vi "Test To Report Entry.vi"(8 "error in (no error)":errorcluster, 10 "Test Node":T1) -> (0 "error out":errorcluster, 2 "String":string)   [LabVIEW 2013, in "Caraya.lvlib" / "Test Report.Event.lvclass"]
uses:
  Test Report.Event.lvclass
  Test Result/Test Node (Extended).ctl
  Test Result/Test Registration Data.ctl
  Test Report/Test Report.lvclass
  Test Result/Test Result.lvclass
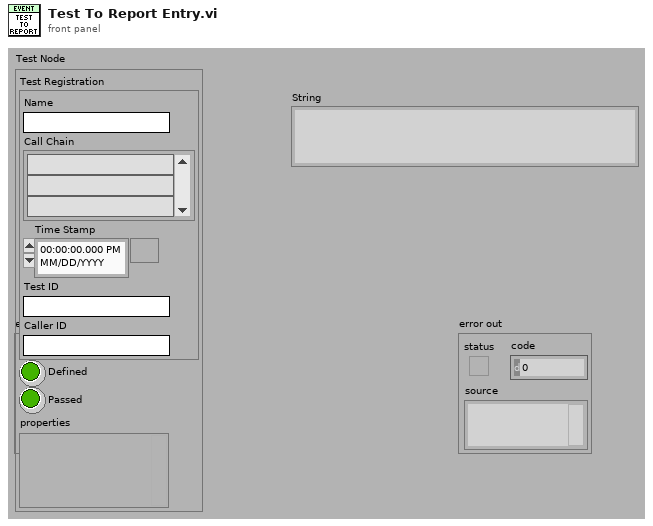
[diagram p1: front panel]
types:
  T1 = typedef "Caraya.lvlib/Test Result.lvclass/Test Node (Extended).ctl" = cluster{"Test Registration":T2, "Defined":bool, "Passed":bool, "properties":variant}
  T2 = typedef "Caraya.lvlib/Test Result.lvclass/Test Registration Data.ctl" = cluster{"Name":string, "Call Chain":string[], "Time Stamp":timestamp, "Test ID":string, "Caller ID":string}
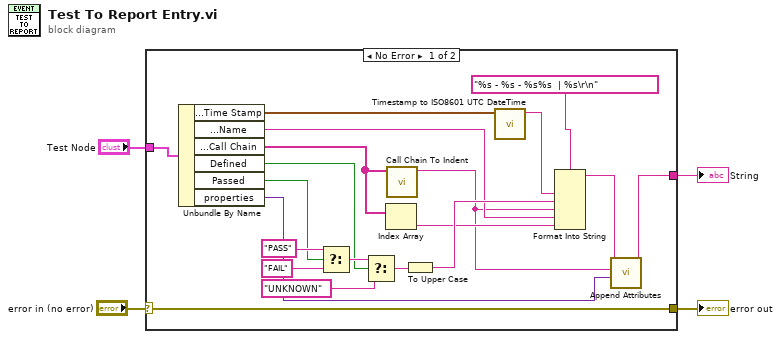
[diagram p0: block diagram]
diagram:
  n1 = case shown="No Error" "error in (no error)" {
    selector: "error in (no error)" -> [w11 w25]
    tunnel: [w11 w25] -> w3
    tunnel: "Test Node" -> [w24 _]
    tunnel: [w7 _] -> w1
    frame No Error {
      n2 = Unbundle By Name(w24) -> ("Test Registration.Time Stamp"=w10:timestamp, "Test Registration.Name"=w20:string, "Test Registration.Call Chain"=w21:string[], "Defined"=w14:bool, "Passed"=w16:bool, "properties"=w5:variant)
      n3 = Select(t="PASS" ("format string"), s=w16, f="FAIL" ("format string")) -> (s? t:f=w18:string)
      n4 = Select(t=w18, s=w14, f="UNKNOWN" ("format string")) -> (s? t:f=w13:string)
      n5 = Index Array(array=w21) -> (element=w19:string)  [unwired: 1 in]
      n6 = call "Call Chain To Indent.vi"("Call Chain"=w21) -> ("Indent"=w6:string)  [unwired: 10 in]
      n7 = To Upper Case(1:w13) -> (0:w22:string)
      n8 = call <vilib>:"Timestamp to ISO8601 UTC DateTime.vi"("Timestamp (now)"=w10) -> ("ISO8601 UTC DateTime"=w12:string)  [unwired: 10 in]
      n9 = Format Into String(format string="%s - %s - %s%s  | %s\r\n", w12, w22, w6, w20, w19) -> (resulting string=w8:string)  [unwired: 2 in, 1 out]
      n10 = call "Append Attributes.vi"("attributes"=w5, "Indent"=w6, "String in"=w8) -> ("String out"=w7:string)  [unwired: 7 in, 1 out]
    }
    frame Error {
    }
  }
  "error out" <- w3
  "String" <- w1
